vi "labview.vi"() -> ()   [LabVIEW 2015]
uses:
  <vilib>/Utility/file.llb/Write Delimited Spreadsheet (DBL).vi
panel:
  in  "stop":bool
  in  "ESP_START":dbl
  out "dt 2":dbl
  in  "STOP":dbl
  in  "START ESP32":bool
  out "dt":dbl
  in  "stop 2":bool
  in  "START":bool
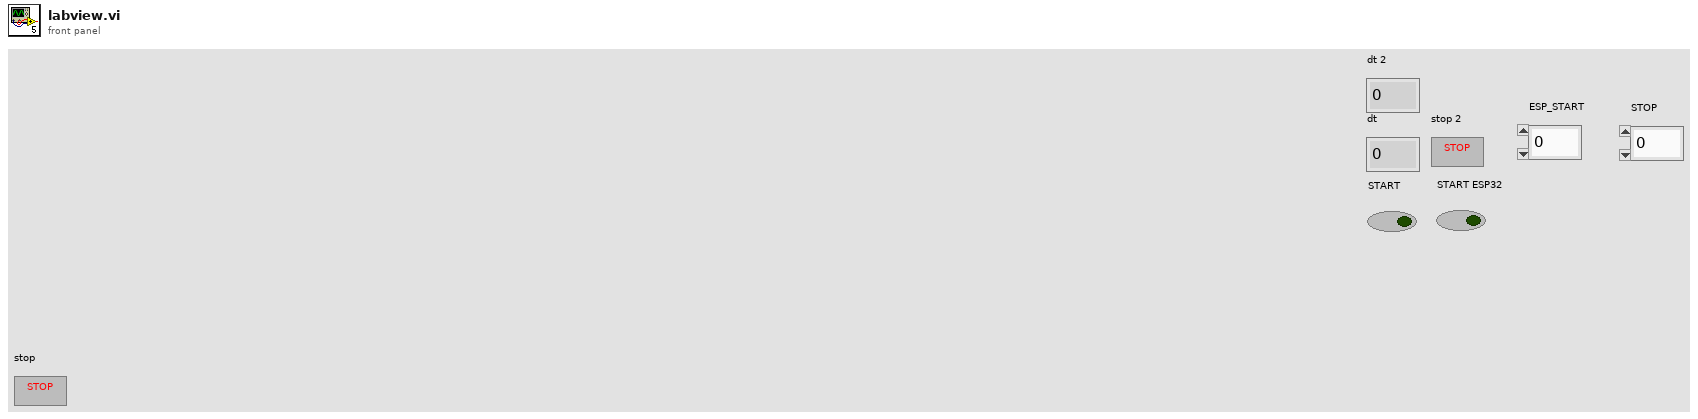
[diagram p1: front panel]
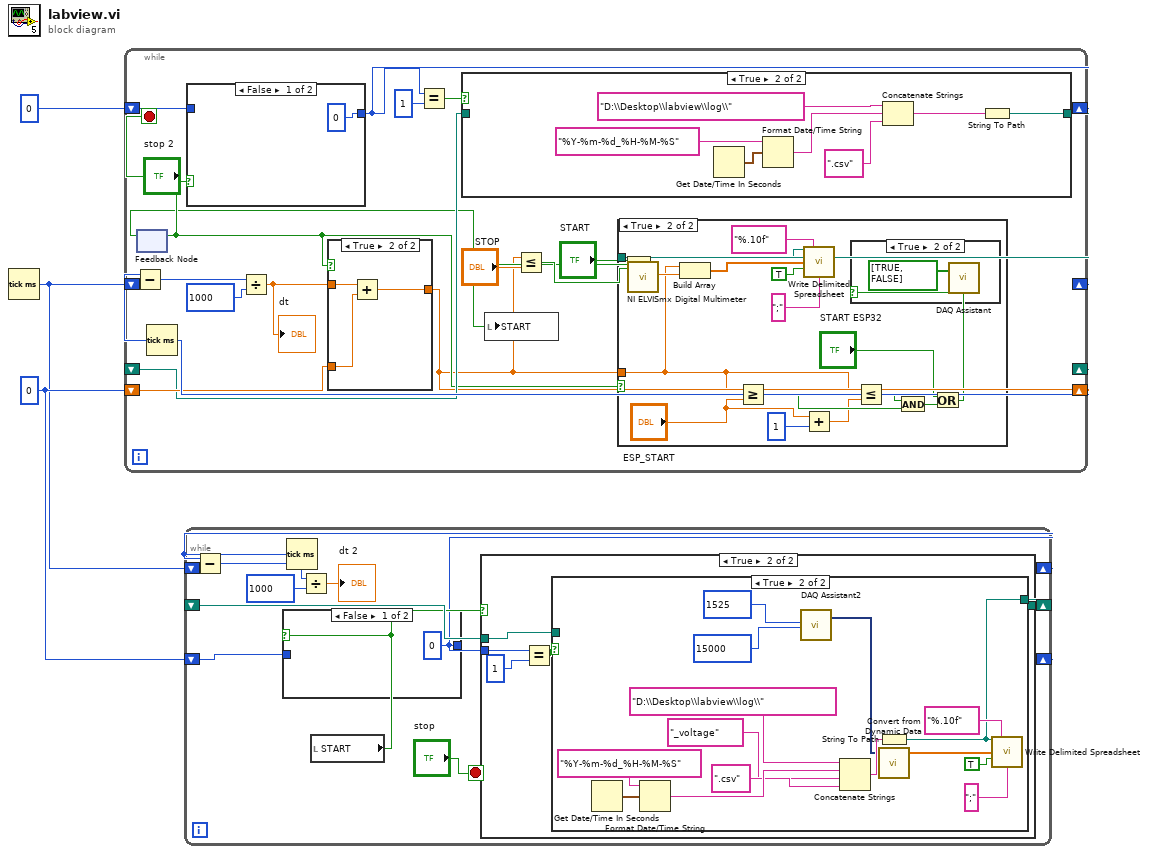
[diagram p0: block diagram]
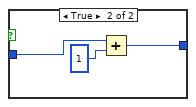
[diagram p4: hidden frame]
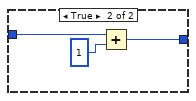
[diagram p5: hidden frame]
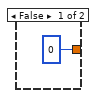
[diagram p7: hidden frame]
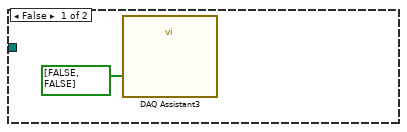
[diagram p8: hidden frame]
diagram:
  w2 = 0
  n1 = Tick Count (ms)() -> (millisecond timer value=w1:u32)
  n2 = while {
    shift-right: [w20] -> _
    shift-left: w1 -> [w21]
    shift-right: [w4] -> _
    shift-left: w2 -> [w17]
    shift-right: [w15] -> _
    shift-left: 0 -> [w16]
    shift-right: [w6] -> _
    shift-left: _ -> [w12]
    stop <- "stop 2" stop-if-true
    n3 = feedback #1() -> (w7:bool)  [unwired: 1 in]
    n4 = Tick Count (ms)() -> (millisecond timer value=w20:u32)
    n5 = Subtract(x=w20, y=w21) -> (x-y=w19:u32)
    n6 = case shown="False" w7 {
      tunnel: w16 -> [_ w26]
      tunnel: [0 w25] -> w15
      frame False {
      }
      frame True {
        n7 = Add(x=w26, y=1) -> (x+y=w25:i32)
      }
    }
    n8 = Divide(x=w19, y=1000) -> (x/y=w11:dbl)
    "dt" <- w11
    n9 = case shown="True" w7 {
      tunnel: w17 -> [_ w38]
      tunnel: w11 -> [_ w37]
      tunnel: [0 w36] -> w4
      frame False {
      }
      frame True {
        n10 = Add(x=w37, y=w38) -> (x+y=w36:dbl)
      }
    }
    n11 = Equal?(x=w15, y=1) -> (x = y?=w13:bool)
    n12 = case shown="True" w13 {
      tunnel: [w27 w29] -> w6
      tunnel: w12 -> [w27 _]
      frame False {
      }
      frame True {
        n13 = Get Date/Time In Seconds() -> (seconds since 1Jan1904=w30:timestamp)
        n14 = Format Date/Time String(time format string (%c)="%Y-%m-%d_%H-%M-%S", seconds (now)=w30) -> (date/time string=w33:string)  [unwired: 1 in]
        n15 = Concatenate Strings("D:\\Desktop\\labview\\log\\", w33, ".csv") -> (w31:string)
        n16 = String To Path(string=w31) -> (path=w29:path)
      }
    }
    n17 = Less Or Equal?(x=w4, y="STOP") -> (x <= y?=w10:bool)
    n18 = case shown="True" w7 {
      tunnel: w4 -> [_ w46]
      tunnel: w6 -> [_ w44]
      frame False {
        n19 = call "DAQ Assistant3"("data"=bool[] [FALSE, FALSE]) -> ()  [unwired: 17 in, 2 out]
      }
      frame True {
        n20 = call "NI ELVISmx Digital Multimeter"() -> ("Measurement"=w47:dbl)  [unwired: 17 in, 2 out]
        n21 = Build Array(w46, w47) -> (w41:dbl[])
        n22 = Greater Or Equal?(x=w46, y="ESP_START") -> (x >= y?=w51:bool)
        n23 = call-poly <vilib>:"Write Delimited Spreadsheet.vi"("file path (dialog if empty)"=w44, "format (%.3f)"="%.10f", "1D data"=w41, "append to file? (F)"=TRUE, "delimiter (\\t)"=";") -> ()  [unwired: 9 in, 2 out]
        n24 = Add(x="ESP_START", y=1) -> (x+y=w48:dbl)
        n25 = Less Or Equal?(x=w46, y=w48) -> (x <= y?=w52:bool)
        n26 = And(x=w52, y=w51) -> (x .and. y?=w53:bool)
        n27 = Or(x="START ESP32", y=w53) -> (x .or. y?=w40:bool)
        n28 = case shown="True" w40 {
          frame False {
          }
          frame True {
            n29 = call "DAQ Assistant"("data"=bool[] [TRUE, FALSE]) -> ()  [unwired: 17 in, 2 out]
          }
        }
      }
    }
    n30 = And(x="START", y=w10) -> (x .and. y?=w5:bool)
    n31 = feedback-in #1(w5) -> ()
    n32 = local write "START"(w5) -> ()
  }
  n33 = while {
    shift-right: [w57] -> _
    shift-left: w2 -> [w58]
    shift-right: [w61] -> _
    shift-left: _ -> [w60]
    shift-right: [w66] -> _
    shift-left: w1 -> [w65]
    stop <- "stop" stop-if-true
    n34 = Tick Count (ms)() -> (millisecond timer value=w66:u32)
    n35 = Subtract(x=w66, y=w65) -> (x-y=w64:u32)
    n36 = Divide(x=w64, y=1000) -> (x/y=→"dt 2":dbl)
    n37 = local read "START"() -> (w59:bool)
    n38 = case shown="False" w59 {
      tunnel: w58 -> [_ w91]
      tunnel: [0 w90] -> w57
      frame False {
      }
      frame True {
        n39 = Add(x=w91, y=1) -> (x+y=w90:i32)
      }
    }
    n40 = case shown="True" w59 {
      tunnel: [w67 w70] -> w61
      tunnel: w60 -> [w67 w69]
      tunnel: w57 -> [_ w68]
      frame False {
      }
      frame True {
        n41 = Equal?(x=w68, y=1) -> (x = y?=w71:bool)
        n42 = case shown="True" w71 {
          tunnel: [w73 w79] -> w70
          tunnel: w69 -> [w73 _]
          frame False {
          }
          frame True {
            n43 = Get Date/Time In Seconds() -> (seconds since 1Jan1904=w85:timestamp)
            n44 = Format Date/Time String(time format string (%c)="%Y-%m-%d_%H-%M-%S", seconds (now)=w85) -> (date/time string=w84:string)  [unwired: 1 in]
            n45 = call "DAQ Assistant2"("rate"=1525, "number of samples"=15000) -> ("data"=w75:dynamicdata)  [unwired: 15 in, 2 out]
            n46 = Concatenate Strings("D:\\Desktop\\labview\\log\\", w84, "_voltage", ".csv") -> (w86:string)
            n47 = String To Path(string=w86) -> (path=w79:path)
            n48 = call "Convert from Dynamic Data"("Dynamic Data Type"=w75) -> ("Array"=w74:dbl[])  [unwired: 3 in]
            n49 = call-poly <vilib>:"Write Delimited Spreadsheet.vi"("file path (dialog if empty)"=w79, "format (%.3f)"="%.10f", "1D data"=w74, "append to file? (F)"=TRUE, "delimiter (\\t)"=";") -> ()  [unwired: 9 in, 2 out]
          }
        }
      }
    }
  }
